vi "Tusk.SystemErrorLogger.vi"(8 "error in (no error)":errorcluster, 11 "Tusk in":refnum<class "Tusk.lvclass">) -> (0 "error out":errorcluster, 3 "Tusk out":refnum<class "Tusk.lvclass">)   [LabVIEW 2018, in "Application.lvlib" / "Tusk.lvclass"]
uses:
  Tusk.lvclass
  Tusk.lvclass/Tusk.ctl
  <vilib>/Utility/SystemLogging/NI_SystemLogging.lvlib
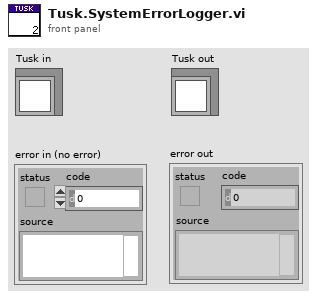
[diagram p1: front panel]
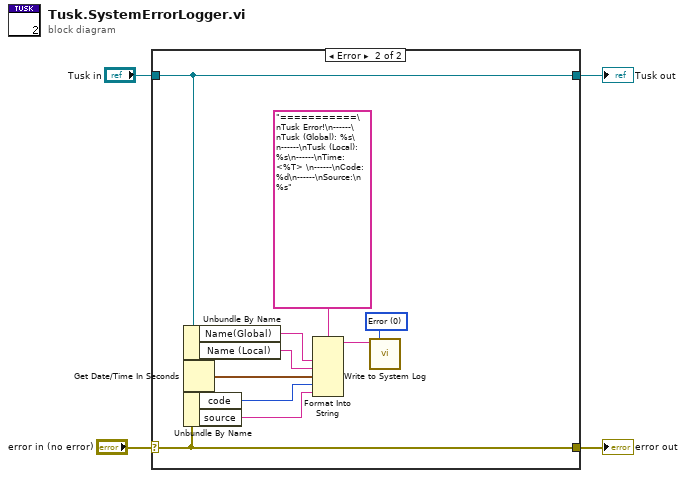
[diagram p0: block diagram]
diagram:
  n1 = case shown="Error" "error in (no error)" {
    selector: "error in (no error)" -> [w6 w9]
    tunnel: [w6 w9] -> w4
    tunnel: [w5 w15] -> w2
    tunnel: "Tusk in" -> [w5 w15]
    frame No Error {
    }
    frame Error {
      w11 = 0 items=["Error", "Warning", "Informational"] ("severity")
      n2 = Unbundle By Name(w15) -> ("Name(Global)"=w14:string, "Name (Local)"=w13:string)
      n3 = Get Date/Time In Seconds() -> (seconds since 1Jan1904=w12:timestamp)
      n4 = Unbundle By Name(w9) -> ("code"=w8:i32, "source"=w7:string)
      n5 = Format Into String(format string="===========\nTusk Error!\n------\nTusk (Global): %s\n------\nTusk (Local): %s\n------\nTime: <%T> \n------\nCode: %d\n------\nSource:\n    %s", w14, w13, w12, w8, w7) -> (resulting string=w10:string)  [unwired: 2 in, 1 out]
      n6 = call <vilib>:"Write to System Log.vi"("severity"=w11, "message"=w10) -> ()  [unwired: 9 in, 1 out]
    }
  }
  "error out" <- w4
  "Tusk out" <- w2
